vi "ComputeXCorXY.vi"(2 "position":cluster{"X":sgl, "Y":sgl}, 3 "iterations":i32=2, 4 "tracker":u64) -> (0 "position":cluster{"X":sgl, "Y":sgl}, 1 "tracker":u64)   [LabVIEW 2011]
uses:
  TrackerDLL.vi
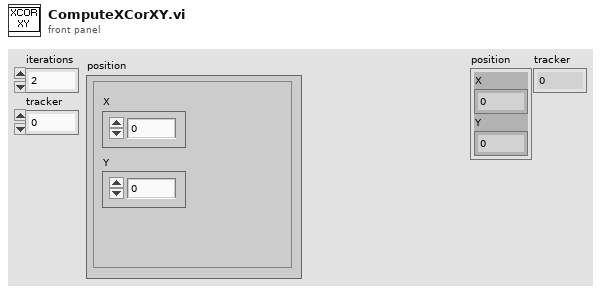
[diagram p1: front panel]
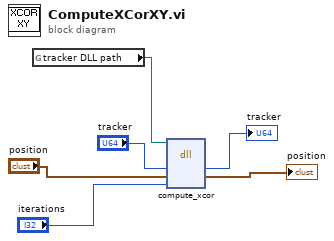
[diagram p0: block diagram]
diagram:
  n1 = global read "TrackerDLL.vi" "tracker DLL path"() -> (w1:path)
  n2 = dll-call lib="D:/jcnossen1/cudaqi-tracker/cudatrack-labview/cputrack.dll" fn="compute_xcor"(path in=w1, "tracker"="tracker", "position"="position", "iterations"="iterations") -> ("tracker"=→"tracker":u64, "position"=→"position":cluster{"X":sgl, "Y":sgl})  [unwired: 4 in, 2 out]
